vi "Defender.vi"(4 "balls":T1[](array[typedef]), 6 "geometry":T2, 9 "Numeric":i32, 10 "Robot":T3, 11 "command\nenum":T4) -> (2 "output cluster":T3)   [LabVIEW 2016]
uses:
  Core/AI Robot.ctl
  Command Enum.ctl
  Core/Field Size.ctl
  Core/AI Ball.ctl
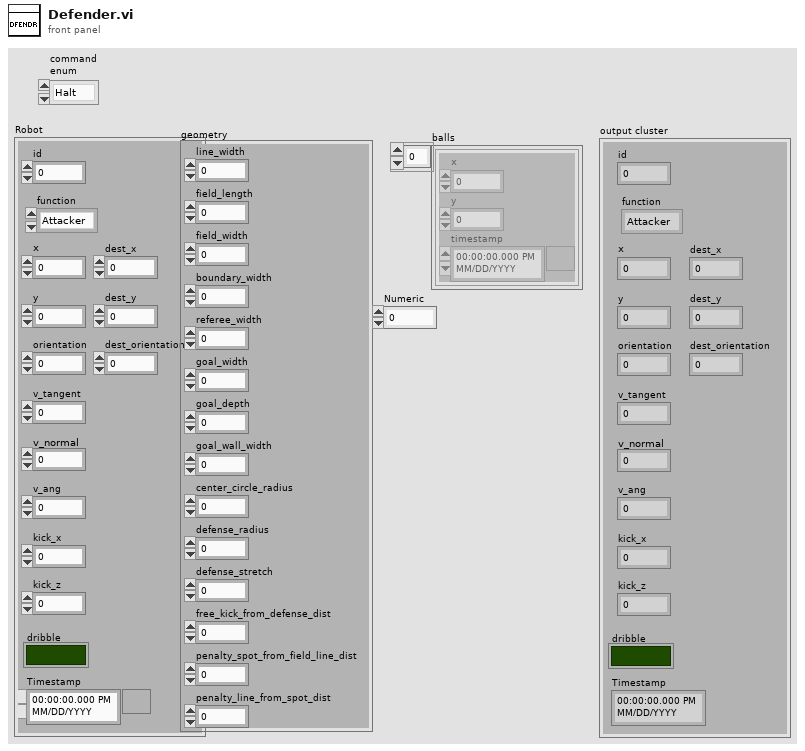
[diagram p1: front panel]
types:
  T1 = typedef "AI Ball.ctl" = cluster{"x":dbl, "y":dbl, "timestamp":timestamp}
  T2 = typedef "Field Size.ctl" = cluster{"line_width":u32, "field_length":u32, "field_width":u32, "boundary_width":u32, "referee_width":u32, "goal_width":u32, "goal_depth":u32, "goal_wall_width":u32, "center_circle_radius":u32, "defense_radius":u32, "defense_stretch":u32, "free_kick_from_defense_dist":u32, "penalty_spot_from_field_line_dist":u32, "penalty_line_from_spot_dist":u32}
  T3 = typedef "AI Robot.ctl" = cluster{"id":u32, "function":enum16{"Attacker", "Goalie", "Defender"}, "x":dbl, "y":dbl, "orientation":dbl, "v_tangent":dbl, "v_normal":dbl, "v_ang":dbl, "kick_x":dbl, "kick_z":dbl, "dribble":bool, "Timestamp":timestamp, "dest_x":dbl, "dest_y":dbl, "dest_orientation":dbl}
  T4 = typedef "Command Enum.ctl" = enum16{"Halt", "Stop", "Force Start", "PKA Normal Start", "Prepare Kickoff Ally", "PKE Normal Start", "Prepare Kickoff Enemy", "Prepare Penalty Ally", "Penalty Ally", "Prepare Penalty Enemy", "Penalty Enemy", "Direct Free Enemy", "Direct Free Ally", "Indirect Free Enemy", "Indirect Free Ally", "Timeout Enemy", "Timeout Ally", "Goal Enemy", "Goal Ally", "Ball Placement Enemy", "Ball Placement Ally", "None"}
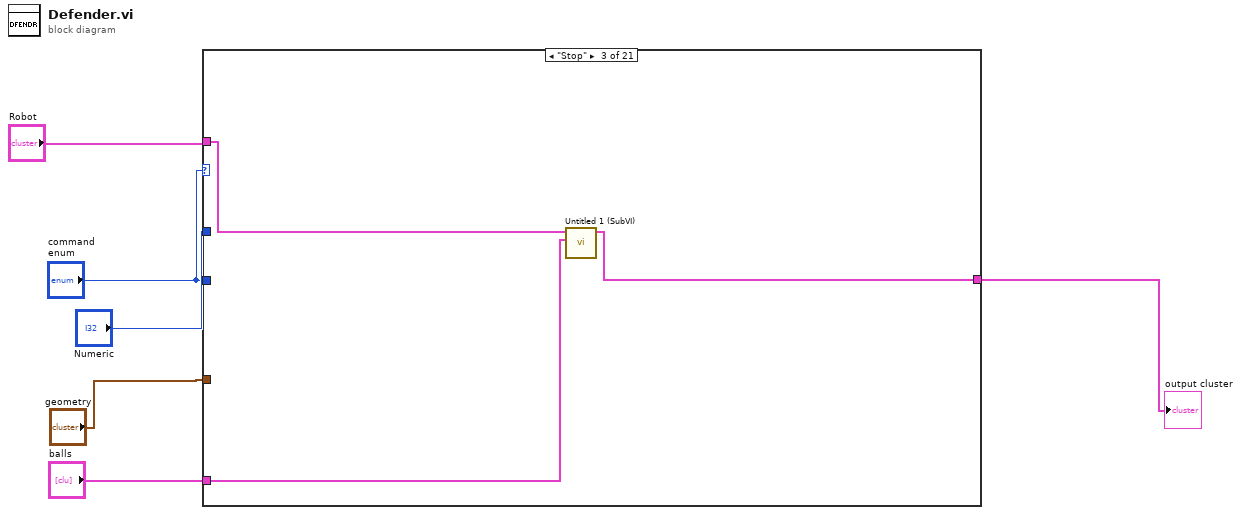
[diagram p0: block diagram]
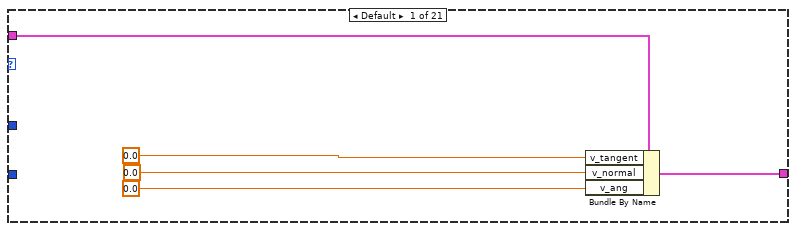
[diagram p2: hidden frame]
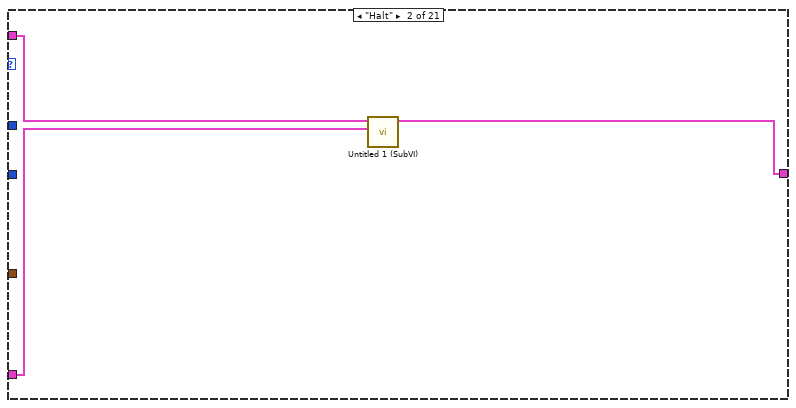
[diagram p3: hidden frame]
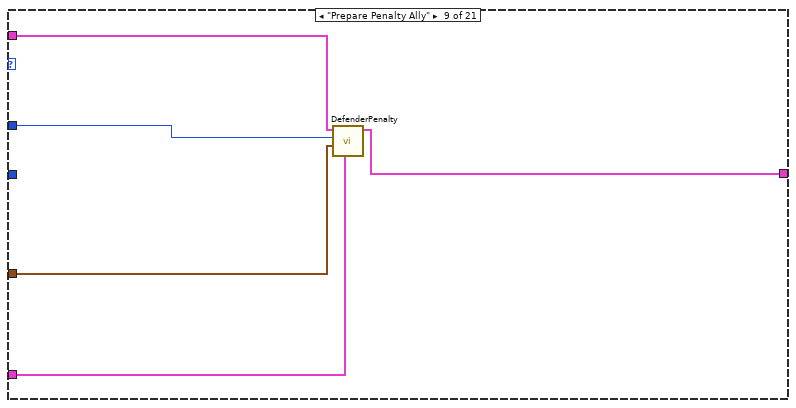
[diagram p9: hidden frame]
diagram:
  n1 = case shown="\"Stop\"" "command\nenum" {
    tunnel: "Robot" -> [w11 w13 w16 w18 w19 w20 w21 w22 w27 w28 w29 w30 w31 w32 w33 w34 w35 w36 w37 w38 w39]
    tunnel: [w7 w12 w15 w18 w19 w20 w21 w22 w23 w28 w29 w30 w31 w32 w33 w34 w35 w36 w37 w38 w39] -> w6
    tunnel: "balls" -> [_ w14 w17 _ _ _ _ _ w24 _ _ _ _ _ _ _ _ _ _ _ _]
    tunnel: "geometry" -> [_ _ _ _ _ _ _ _ w25 _ _ _ _ _ _ _ _ _ _ _ _]
    tunnel: "Numeric" -> [_ _ _ _ _ _ _ _ w26 _ _ _ _ _ _ _ _ _ _ _ _]
    tunnel: "command\nenum" -> [_ _ _ _ _ _ _ _ _ _ _ _ _ _ _ _ _ _ _ _ _]
    frame Default {
      n2 = Bundle By Name(cluster=w11, "v_tangent"=0.0 ("v_x"), "v_normal"=0.0 ("v_y"), "v_ang"=0.0) -> (w7:T3)
    }
    frame "Halt" {
      n3 = call "Untitled 1 (SubVI).vi"("balls"=w14, "Robot in"=w13) -> ("Robot out"=w12:T3)  [unwired: 9 in]
    }
    frame "Stop" {
      n4 = call "Untitled 1 (SubVI).vi"("balls"=w17, "Robot in"=w16) -> ("Robot out"=w15:T3)  [unwired: 9 in]
    }
    frame "Force Start" {
    }
    frame "PKA Normal Start" {
    }
    frame "Prepare Kickoff Ally" {
    }
    frame "PKE Normal Start" {
    }
    frame "Prepare Kickoff Enemy" {
    }
    frame "Prepare Penalty Ally" {
      n5 = call "DefenderPenalty.vi"("balls"=w24, "Field Size in"=w25, "Numeric"=w26, "Robot in"=w27) -> ("Robot out"=w23:T3)  [unwired: 7 in]
    }
    frame "Prepare Penalty Enemy" {
    }
    frame "Direct Free Enemy" {
    }
    frame "Direct Free Ally" {
    }
    frame "Indirect Free Enemy" {
    }
    frame "Indirect Free Ally" {
    }
    frame "Timeout Enemy" {
    }
    frame "Timeout Ally" {
    }
    frame "Goal Enemy" {
    }
    frame "Goal Ally" {
    }
    frame "Ball Placement Enemy" {
    }
    frame "Ball Placement Ally" {
    }
    frame "None" {
    }
  }
  "output cluster" <- w6
